vi "DAC Configure.vi"(8 "error in":errorcluster, 11 "DAC Keller BNC in":refnum<class "DAC Keller BNC.lvclass">) -> (0 "error out":errorcluster, 3 "DAC Keller BNC out":refnum<class "DAC Keller BNC.lvclass">)   [LabVIEW 2019, in "DAC.lvlib" / "DAC Keller BNC.lvclass"]
uses:
  DAC Keller BNC.lvclass
  C:/Users/wg/Documents/LV_Projects/test-stand/App/DAC/DAC.lvclass
  DAC.lvclass/DAC.ctl
  DAC Keller BNC.lvclass/DAC Keller BNC.ctl
  <vilib>/DAQmx/create/channels.llb/DAQmx Create Channel (AI-Voltage-Basic).vi
  <vilib>/DAQmx/configure/timing.llb/DAQmx Timing (Sample Clock).vi
  DAC.lvclass
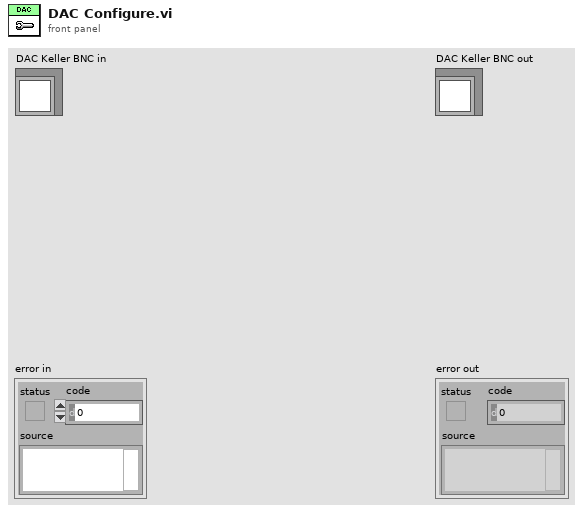
[diagram p1: front panel]
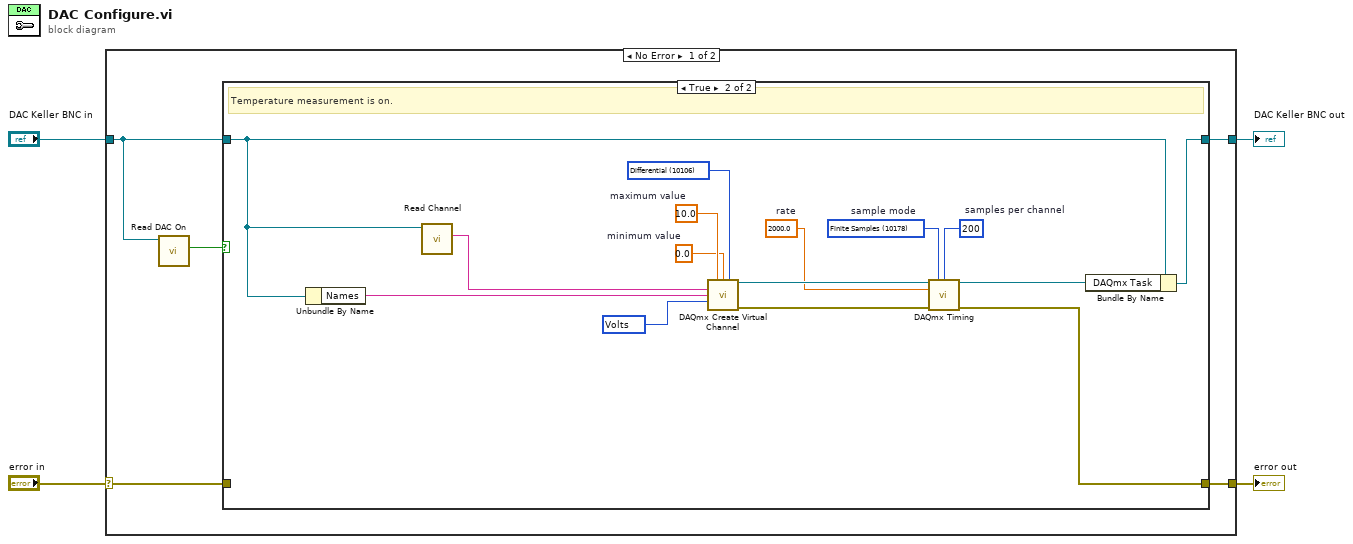
[diagram p0: block diagram]
diagram:
  n1 = case shown="No Error" "error in" {
    selector: "error in" -> [w6 w28]
    tunnel: [w5 w28] -> w4
    tunnel: [w7 w27] -> w3
    tunnel: "DAC Keller BNC in" -> [w9 w27]
    frame No Error {
      n2 = call "Read DAC On.vi"("DAC in"=w9) -> ("DAC On"=w8:bool)  [unwired: 8 in, 2 out]
      n3 = case shown="True" w8 {
        tunnel: w9 -> [w11 w24]
        tunnel: [w11 w26] -> w7
        tunnel: w6 -> [w10 _]
        tunnel: [w10 w18] -> w5
        frame False {
          # "Temperature measurement is off."
        }
        frame True {
          w12 = 10106 items=["Default"=-1, "RSE"=10083, "NRSE"=10078, "Differential"=10106, "Pseudodifferential"=12529] ("input terminal configuration")
          w13 = 0.0  # minimum value
          w14 = 10.0  # maximum value
          w15 = 200  # samples per channel
          w16 = 2000.0  # rate
          w17 = 10178 items=["Finite Samples"=10178, "Continuous Samples"=10123, "Hardware Timed Single Point"=12522]  # sample mode
          w22 = 10348 items=["Volts"=10348, "From Custom Scale"=10065] ("units")
          # "Temperature measurement is on."
          n4 = Unbundle By Name(w24) -> ("Names"=w25:string)
          n5 = call "Read Channel.vi"("DAC in"=w24) -> ("Channel"=w23:string)  [unwired: 8 in, 2 out]
          n6 = call-poly <vilib>:"DAQmx Create Virtual Channel.vi"("maximum value"=w14, "minimum value"=w13, "input terminal configuration"=w12, "physical channels"=w23, "name to assign"=w25, "units"=w22) -> ("task out"=w21:refnum<k21>, "error out"=w20:errorcluster)  [unwired: 8 in]
          n7 = call-poly <vilib>:"DAQmx Timing.vi"("task/channels in"=w21, "sample mode"=w17, "samples per channel"=w15, "rate"=w16, "error in"=w20) -> ("task out"=w19:refnum<k21>, "error out"=w18:errorcluster)  [unwired: 9 in]
          n8 = Bundle By Name(cluster=w24, "DAQmx Task"=w19) -> (w26:refnum<class "DAC Keller BNC.lvclass">)
        }
      }
    }
    frame Error {
    }
  }
  "error out" <- w4
  "DAC Keller BNC out" <- w3
